vi "FMA1600A Dryer Data Build.vi"(7 "Barometric Pressure.Barometric Pressure (in. Hg)":dbl, 8 "Error In":errorcluster, 11 "DAQ Data In in":T1) -> (0 "Error Out":errorcluster, 2 "LPM (Vol. Flow)":dbl, 3 "Dryer Data":string[][](array[string]))   [LabVIEW 2018]
uses:
  Trunk/Range/Type Definitions/RANGE DAQ Data Four Meters.ctl
  Trunk/Range/Type Definitions/RANGE DAQ Data.ctl
  Type Definitions/FMA1600A Gas Type.ctl
  Type Definitions/FMA1600A Units String.ctl
  Trunk/Range/Type Definitions/RANGE GAS Data.ctl
  Trunk/Range/Type Definitions/RANGE Panel Data.ctl
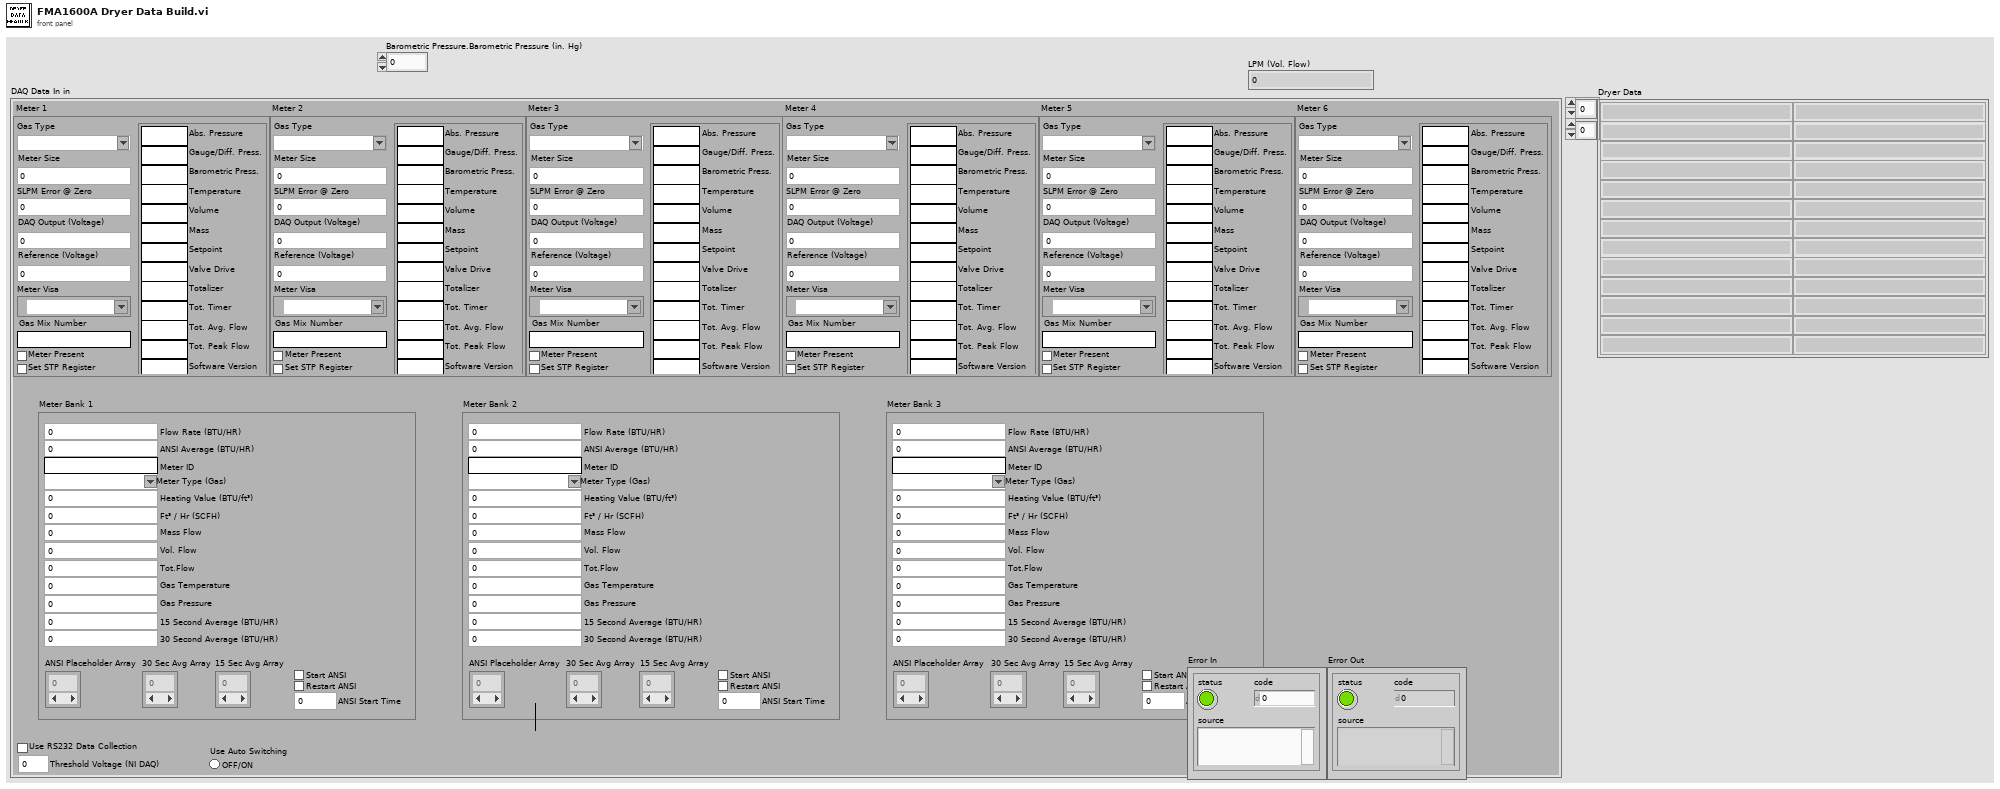
[diagram p1: front panel]
types:
  T1 = typedef "RANGE DAQ Data Four Meters.ctl" = cluster{"Meter 1":T2, "Meter 2":T2, "Meter 3":T2, "Meter 4":T2, "Meter 5":T2, "Meter 6":T2, "Meter Bank 1":T5, "Meter Bank 2":T5, "Meter Bank 3":T5, "Threshold Voltage (NI DAQ)":dbl, "Use RS232 Data Collection":bool, "Use Auto Switching":bool}
  T2 = typedef "RANGE DAQ Data.ctl" = cluster{"Meter Size":dbl, "DAQ Output (Voltage)":dbl, "Reference (Voltage)":dbl, "Meter Present":bool, "Meter Visa":refnum<visa-resource-name>, "Gas Type":T3, "SLPM Error @ Zero":dbl, "Gas Mix Number":string, "Set STP Register":bool, "Measurement Units":T4}
  T3 = typedef "FMA1600A Gas Type.ctl" = string
  T4 = typedef "FMA1600A Units String.ctl" = cluster{"Abs. Pressure":string, "Gauge/Diff. Press.":string, "Barometric Press.":string, "Temperature":string, "Volume":string, "Mass":string, "Setpoint":string, "Valve Drive":string, "Totalizer":string, "Tot. Timer":string, "Tot. Avg. Flow":string, "Tot. Peak Flow":string, "Software Version":string}
  T5 = typedef "RANGE GAS Data.ctl" = cluster{"Flow Rate (BTU/HR)":dbl, "ANSI Placeholder Array":dbl[], "15 Sec Avg Array":dbl[], "30 Sec Avg Array ":dbl[], "ANSI Average (BTU/HR)":dbl, "Panel Data":T6, "Start ANSI":bool, "ANSI Start Time":dbl, "Restart ANSI":bool, "Meter ID":string}
  T6 = typedef "RANGE Panel Data.ctl" = cluster{"Meter Type (Gas)":T3, "Heating Value (BTU/ft³)":dbl, "Ft³ / Hr (SCFH)":dbl, "15 Second Average (BTU/HR)":dbl, "30 Second Average (BTU/HR)":dbl, "Mass Flow":dbl, "Vol. Flow":dbl, "Gas Temperature":dbl, "Gas Pressure":dbl, "Tot.Flow":dbl}
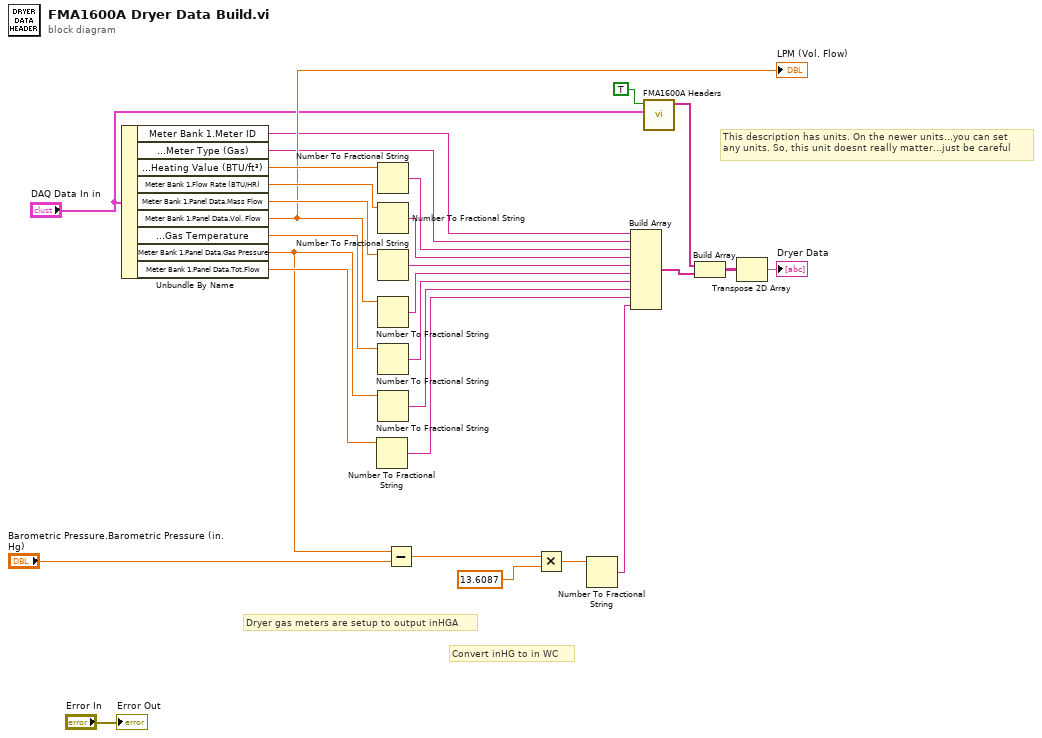
[diagram p0: block diagram]
diagram:
  # "This description has units. On the newer units...you can set\nany units. So, this unit doesnt really matter...just be careful"
  # "Convert inHG to in WC"
  # "Dryer gas meters are setup to output inHGA"
  n1 = Unbundle By Name("DAQ Data In in") -> ("Meter Bank 1.Meter ID"=w1:string, "Meter Bank 1.Panel Data.Meter Type (Gas)"=w3:T3, "Meter Bank 1.Panel Data.Heating Value (BTU/ft³)"=w28:dbl, "Meter Bank 1.Flow Rate (BTU/HR)"=w27:dbl, "Meter Bank 1.Panel Data.Mass Flow"=w26:dbl, "Meter Bank 1.Panel Data.Vol. Flow"=w25:dbl, "Meter Bank 1.Panel Data.Gas Temperature"=w24:dbl, "Meter Bank 1.Panel Data.Gas Pressure"=w9:dbl, "Meter Bank 1.Panel Data.Tot.Flow"=w23:dbl)
  "LPM (Vol. Flow)" <- w25
  n2 = Number To Fractional String(number=w23) -> (F-format string=w16:string)  [unwired: 3 in]
  n3 = Number To Fractional String(number=w28) -> (F-format string=w22:string)  [unwired: 3 in]
  n4 = Number To Fractional String(number=w27) -> (F-format string=w21:string)  [unwired: 3 in]
  n5 = Number To Fractional String(number=w26) -> (F-format string=w20:string)  [unwired: 3 in]
  n6 = Number To Fractional String(number=w25) -> (F-format string=w19:string)  [unwired: 3 in]
  n7 = Number To Fractional String(number=w24) -> (F-format string=w18:string)  [unwired: 3 in]
  n8 = Number To Fractional String(number=w9) -> (F-format string=w17:string)  [unwired: 3 in]
  n9 = Subtract(x=w9, y="Barometric Pressure.Barometric Pressure (in. Hg)") -> (x-y=w7:dbl)
  n10 = Multiply(x=w7, y=13.6087) -> (x*y=w5:dbl)
  n11 = Number To Fractional String(number=w5) -> (F-format string=w4:string)  [unwired: 3 in]
  n12 = Build Array(w1, w3, w22, w21, w20, w19, w18, w17, w16, w4) -> (w15:T3[])
  n13 = call "FMA1600A Headers.vi"("All Meter Data"="DAQ Data In in", "Dryer?"=TRUE) -> ("Range/Dryer Headers 1"=w14:string[])  [unwired: 6 in, 3 out]
  n14 = Build Array(w14, w15) -> (w12:T3[][])
  n15 = Transpose 2D Array(2D array=w12) -> (transposed array=→"Dryer Data":T3[][])
  "Error Out" <- "Error In"
